vi "Check software integrity package.vi"(0 "Package Integrity File Path":path) -> (2 "File list not ok":string, 3 "Package not ok":bool)   [LabVIEW 2010]
uses:
  package/Search 1D Array (Boolean)__ogtk.vi
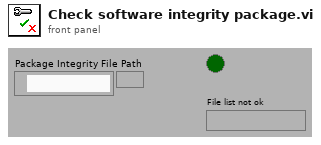
[diagram p1: front panel]
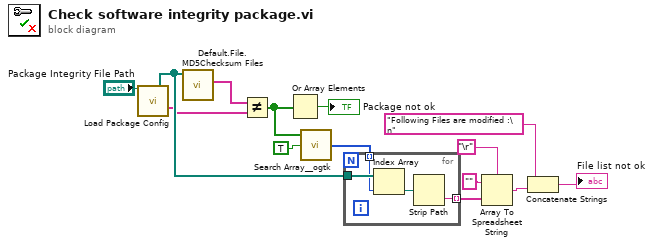
[diagram p0: block diagram]
diagram:
  n1 = call "Load Package Config.vi"("Path"="Package Integrity File Path") -> ("Path Out"=w6:path[], "MD5 Chk sum"=w2:string[])  [unwired: 9 in, 4 out]
  n2 = call "Default.File.MD5Checksum Files.vi"("FilePaths"=w6) -> ("Checksum Array"=w1:string[])  [unwired: 8 in, 2 out]
  n3 = Not Equal?(x=w1, y=w2) -> (x != y?=w13:bool[])
  n4 = Or Array Elements(Boolean array=w13) -> (logical OR=→"Package not ok":bool)
  n5 = call-poly "Search Array__ogtk.vi"("Array"=w13, "Element Data"=TRUE) -> ("Indices of Elements"=w5:i32[])  [unwired: 7 in]
  n6 = for {
    tunnel: w5 -> [w17] mode=indexing
    tunnel: w6 -> [w18]
    tunnel: [w15] -> w7 mode=indexing
    n7 = Index Array(array=w18, index=w17) -> (element=w16:path)
    n8 = Strip Path(path=w16) -> (name=w15:string)  [unwired: 1 out]
  }
  n9 = Array To Spreadsheet String(delimiter (Tab)="\r", array=w7, 3:"" ("format string")) -> (spreadsheet string=w10:string)
  n10 = Concatenate Strings("Following Files are modified :\n" ("string"), w10) -> (→"File list not ok":string)
